vi "Amira Bladder Experiment - Multiple - V1.1.vi"() -> ()   [LabVIEW 2020]
uses:
  <userlib>/KQD LabVIEW User/Serial/Controls/SERIAL PortConfig.ctl
  <userlib>/KQD LabVIEW User/Serial/Controls/SERIAL BaudRate.ctl
  <userlib>/KQD LabVIEW User/Button/STOP.ctl
  <userlib>/Amira UART/Public/TypeDefs/AUART StepDir.ctl
  <userlib>/Amira UART/Amira UART.lvclass
  <userlib>/KQD LabVIEW User/Serial/Serial.lvlib
panel:
  out "Data":dbl[][](graph)
  in  "Stop":T1
  out "Idx":i32
  in  "Iteration":i32
  in  "RunWith":cluster{"Steps":i32, "Rates":i32}={"Steps"=400, "Rates"=40}
  in  "Folder":path=path "C:/Amira Data/Strip"
  in  "Strip":enum16{"Surface", "Blader"}(ring)
  out "FrontOpen":dbl
  out "BackOpen":dbl
  out "FrontClose":dbl
  out "BackClose":dbl
  in  "StartAt":cluster{"Steps":i32, "Rates":i32}={"Steps"=950, "Rates"=200}
  out "Run":dbl[](graph)
  in  "DAQ":tag="Dev1/port0"
  out "UART":string
  in  "ComPort":refnum<visa-resource-name>
  in  "Config":T2={"BaudRate"=enum."460800", "StopBits"=10, "DataBits"=8, "Parity"=enum."None", "FlowControl"=2, "TimeOut"=1000, "TermChar"=10, "ReadTermEn"=TRUE} {"TermChar" format="%.0x"; "FlowControl" items=["None", "XON/XOFF", "RTS/CTS", "XON/XOFF & RTS/CTS", "DTR/DSR", "XON/XOFF & DTR/DSR"]; "DataBits" min=5 max=8 step=1; "StopBits" items=["1.0"=10, "1.5"=15, "2.0"=20]}
  out "ErrOut":errorcluster
  in  "ErrIn":errorcluster
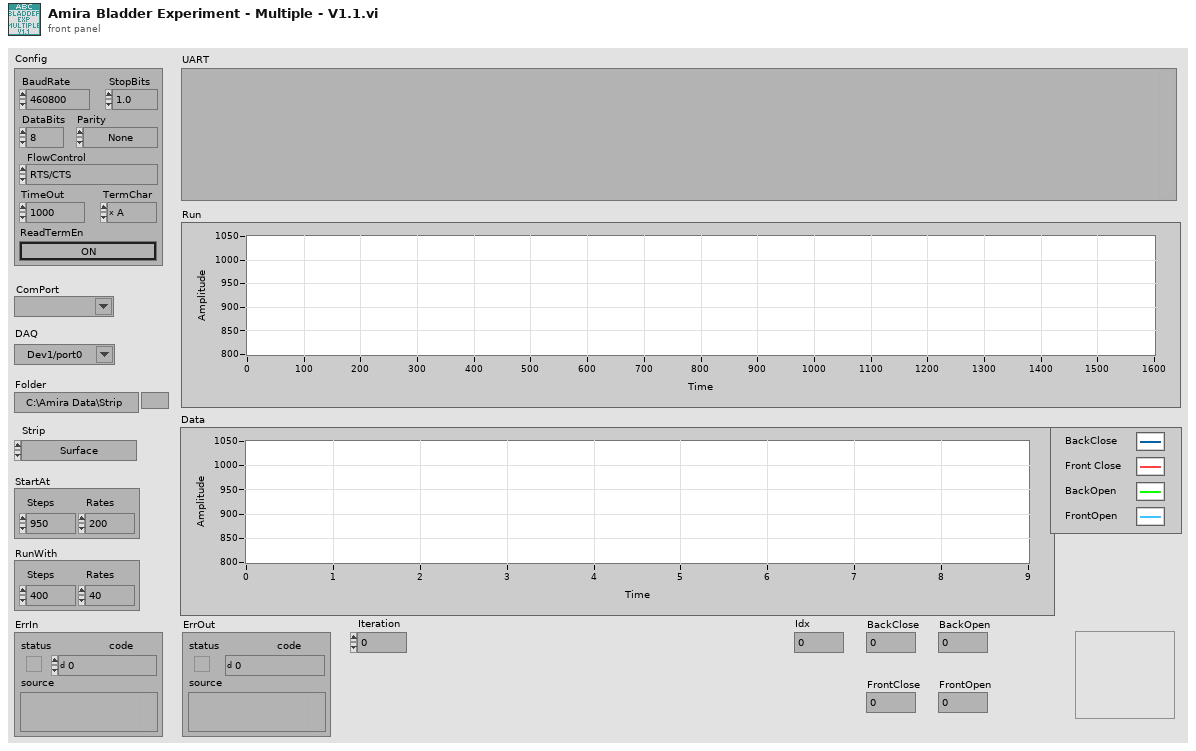
[diagram p1: front panel]
types:
  T1 = typedef "STOP.ctl" = bool
  T2 = typedef "Serial.lvlib/SERIAL PortConfig.ctl" = cluster{"BaudRate":T3, "StopBits":u16, "DataBits":u16, "Parity":enum16{"None", "Odd", "Even", "Mark", "Space"}, "FlowControl":u16, "TimeOut":u32, "TermChar":u8, "ReadTermEn":bool}
  T3 = typedef "SERIAL BaudRate.ctl" = enum16{"2400", "4800", "7200", "9600", "14400", "19200", "28800", "38400", "57600", "115200", "128000", "230400", "460800", "921600"}
  T4 = typedef "Amira UART.lvclass/AUART StepDir.ctl" = enum16{"", "compress", "decompress"}
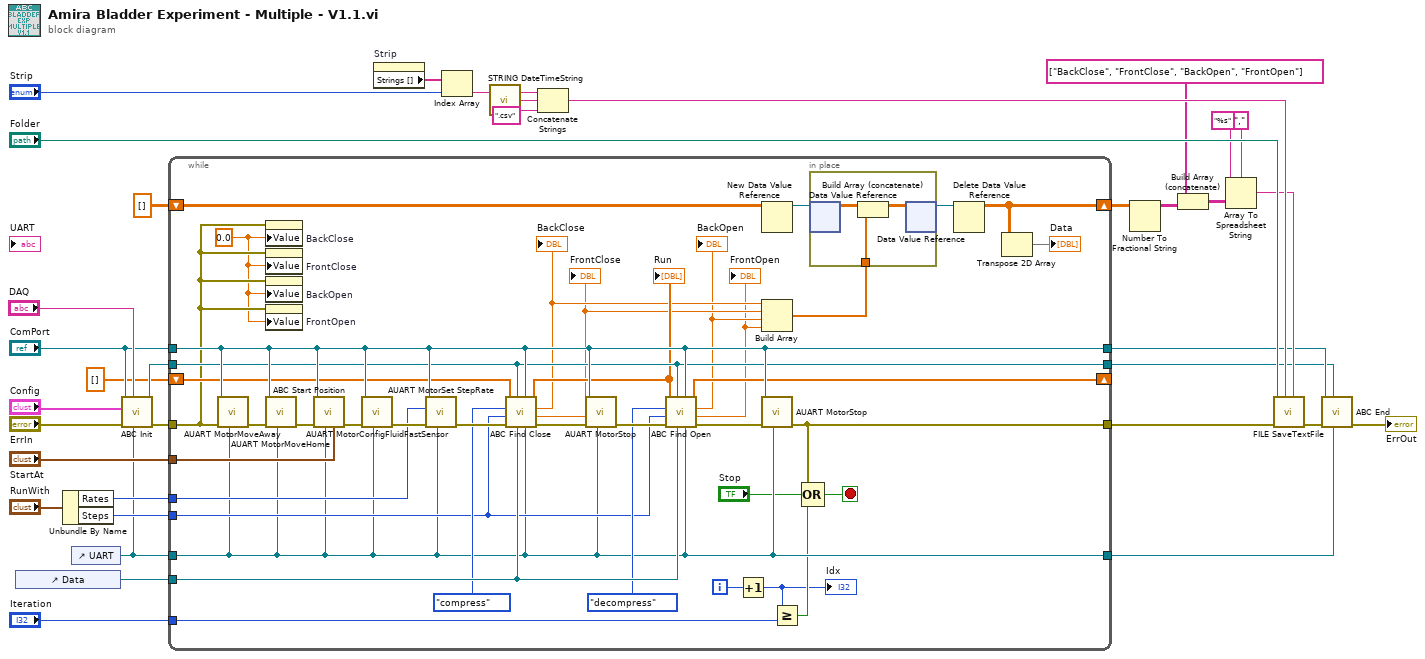
[diagram p0: block diagram]
diagram:
  n1 = control-ref of="Data"() -> (w30:refnum<vi>)
  n2 = Unbundle By Name("RunWith") -> ("Rates"=w16:i32, "Steps"=w15:i32)
  n3 = control-ref of="UART"() -> (w13:refnum<vi>)
  n4 = call "ABC Init.vi"("UART"=w13, "DAQ"="DAQ", "ErrIn"="ErrIn", "PortConfig"="Config", "ComPort"="ComPort") -> ("ErrOut"=w14:errorcluster, "DaqTask"=w31:refnum<k21>)  [unwired: 5 in]
  n5 = while {
    tunnel: "StartAt" -> [w70]
    tunnel: w31 -> [w53]
    tunnel: w30 -> [w66]
    tunnel: w16 -> [w63]
    tunnel: w15 -> [w62]
    tunnel: w13 -> [w60]
    tunnel: "ComPort" -> [w54]
    tunnel: w14 -> [w50]
    tunnel: [w59] -> w11
    tunnel: [w60] -> w8
    tunnel: "Iteration" -> [w57]
    tunnel: [w54] -> w7
    tunnel: [w53] -> w6
    shift-right: [w37] -> w4
    shift-left: dbl[][] [] -> [w39]
    shift-right: [w47] -> _
    shift-left: dbl[] [] ("DataOut") -> [w51]
    i -> [w58]
    stop <- w55 stop-if-true
    w49 = 0.0 ("BackClose")
    n6 = call <userlib>:"AUART MotorMoveAway.vi"("UART"=w60, "ErrIn"=w50, "Port"=w54) -> ("ErrOut"=w61:errorcluster)  [unwired: 8 in]
    n7 = property on="BackClose" class="DigNum (strict)"(error in=w50, "Value"=w49) -> ()  [unwired: 1 in, 2 out]
    n8 = property on="FrontClose" class="DigNum (strict)"(error in=w50, "Value"=w49) -> ()  [unwired: 1 in, 2 out]
    n9 = property on="BackOpen" class="DigNum (strict)"(error in=w50, "Value"=w49) -> ()  [unwired: 1 in, 2 out]
    n10 = property on="FrontOpen" class="DigNum (strict)"(error in=w50, "Value"=w49) -> ()  [unwired: 1 in, 2 out]
    n11 = call <userlib>:"AUART MotorMoveHome.vi"("UART"=w60, "ErrIn"=w61, "Port"=w54) -> ("ErrOut"=w72:errorcluster)  [unwired: 7 in, 1 out]
    n12 = call "ABC Start Position.vi"("Start"=w70, "UART"=w60, "ErrIn"=w72, "ComPort"=w54) -> ("ErrOut"=w71:errorcluster)  [unwired: 6 in, 1 out]
    n13 = call <userlib>:"AUART MotorConfigFluidFastSensor.vi"("UART"=w60, "ErrIn"=w71, "Port"=w54) -> ("ErrOut"=w74:errorcluster)  [unwired: 8 in]
    n14 = call <userlib>:"AUART MotorSet StepRate.vi"("UART"=w60, "ErrIn"=w74, "step_rate"=w63, "Port"=w54) -> ("ErrOut"=w73:errorcluster)  [unwired: 7 in]
    n15 = call "ABC Find Close.vi"("UART"=w60, "ComPort"=w54, "Data"=w66, "DaqTask"=w53, "ErrIn"=w73, "#Step"=w62, "Dir"=AUART_StepDir."compress" ("step_dir"), "DataIn"=w51) -> ("ErrOut"=w69:errorcluster, "FrontClose"=w45:dbl, "BackClose"=w46:dbl, "DataOut"=w52:dbl[])
    "Run" <- w52
    "BackClose" <- w46
    "FrontClose" <- w45
    n16 = call <userlib>:"AUART MotorStop.vi"("UART"=w60, "ErrIn"=w69, "Port"=w54) -> ("ErrOut"=w68:errorcluster)  [unwired: 8 in]
    n17 = call "ABC Find Open.vi"("UART"=w60, "ComPort"=w54, "Data"=w66, "DaqTask"=w53, "ErrIn"=w68, "#Step"=w62, "Dir"=AUART_StepDir."decompress" ("step_dir"), "DataIn"=w52) -> ("ErrOut"=w67:errorcluster, "FrontOpen"=w43:dbl, "BackOpen"=w44:dbl, "DataOut"=w47:dbl[])
    "BackOpen" <- w44
    "FrontOpen" <- w43
    n18 = Increment(x=w58) -> (x+1=w36:i32)
    "Idx" <- w36
    n19 = New Data Value Reference(data value=w39) -> (data value reference=w40:refnum<data-value>)  [unwired: 1 in, 1 out]
    n20 = Build Array(w46, w45, w44, w43) -> (w38:dbl[])
    n21 = call <userlib>:"AUART MotorStop.vi"("UART"=w60, "ErrIn"=w67, "Port"=w54) -> ("ErrOut"=w59:errorcluster)  [unwired: 8 in]
    n22 = Greater Or Equal?(x=w36, y=w57) -> (x >= y?=w56:bool)
    n23 = Compound Arithmetic op=OR(w59, "Stop", w56) -> (w55:T1)
    n24 = in-place {
      in-place-border: w38 -> [w75]
      n25 = in-place-dvr #1(w40) -> (w77:dbl[][])  [unwired: 1 out]
      n26 = Build Array (concatenate)(w77, w75) -> (w76:dbl[][])
      n27 = in-place-dvr #1(w76) -> (w41:refnum<data-value>)  [unwired: 1 out]
    }
    n28 = Delete Data Value Reference(data value reference=w41) -> (data value=w37:dbl[][])  [unwired: 1 in, 1 out]
    n29 = Transpose 2D Array(2D array=w37) -> (transposed array=→"Data":dbl[][])
  }
  n30 = property on="Strip" class="Enum (strict)"() -> ("Strings []"=w29:string[])  [unwired: 2 in, 2 out]
  n31 = Index Array(array=w29, index="Strip") -> (element=w27:string)
  n32 = call <userlib>:"STRING DateTimeString.vi"() -> ("DateTimeStr"=w26:string)  [unwired: 2 in]
  n33 = Concatenate Strings(w27, w26, ".csv" ("string")) -> (w23:string)
  n34 = Number To Fractional String(number=w4) -> (F-format string=w2:string[][])  [unwired: 3 in]
  n35 = Build Array (concatenate)(string[] ["BackClose", "FrontClose", "BackOpen", "FrontOpen"], w2) -> (w21:string[][])
  n36 = Array To Spreadsheet String(delimiter (Tab)=",", array=w21, 3:"%s" ("format string")) -> (spreadsheet string=w19:string)
  n37 = call <userlib>:"FILE SaveTextFile.vi"("Data"=w19, "File"=w23, "ErrIn"=w11, "Folder"="Folder") -> ("ErrOut"=w10:errorcluster)  [unwired: 7 in]
  n38 = call "ABC End.vi"("UART"=w8, "DaqTask"=w6, "ErrIn"=w10, "ComPort"=w7) -> ("ErrOut"=→"ErrOut":errorcluster)  [unwired: 7 in]
